vi "FixStyle.vi"(11 "Control in":refnum<class "Control.lvclass">) -> (3 "Control out":refnum<class "Control.lvclass">)   [LabVIEW 2014, in "Control.lvclass"]
uses:
  Control.lvclass
  Control.lvclass/Control.ctl
  Generic/Generic.lvclass/Generic.ctl
  Generic/Generic.lvclass
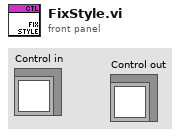
[diagram p1: front panel]
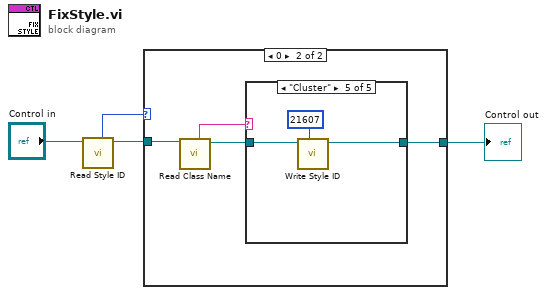
[diagram p0: block diagram]
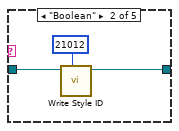
[diagram p4: hidden frame]
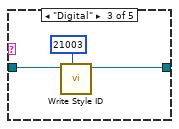
[diagram p5: hidden frame]
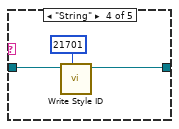
[diagram p6: hidden frame]
diagram:
  n1 = call "Read Style ID.vi"("Control in"="Control in") -> ("Control out"=w2:refnum<class "Control.lvclass">, "Style ID"=w3:u32)  [unwired: 7 in]
  n2 = case shown="0" w3 {
    tunnel: w2 -> [w5 w9]
    tunnel: [w5 w6] -> w1
    frame Default {
    }
    frame 0 {
      n3 = call "Read Class Name.vi"("Generic in"=w9) -> ("Generic out"=w7:refnum<class "Control.lvclass">, "Class Name"=w8:string)  [unwired: 7 in]
      n4 = case shown="\"Cluster\"" w8 {
        tunnel: w7 -> [w10 w13 w16 w19 w22]
        tunnel: [w10 w12 w15 w18 w21] -> w6
        frame Default {
        }
        frame "Boolean" {
          n5 = call "Write Style ID.vi"("Style ID"=u32 21012, "Control in"=w13) -> ("Control out"=w12:refnum<class "Control.lvclass">)  [unwired: 7 in]
        }
        frame "Digital" {
          n6 = call "Write Style ID.vi"("Style ID"=u32 21003, "Control in"=w16) -> ("Control out"=w15:refnum<class "Control.lvclass">)  [unwired: 7 in]
        }
        frame "String" {
          n7 = call "Write Style ID.vi"("Style ID"=u32 21701, "Control in"=w19) -> ("Control out"=w18:refnum<class "Control.lvclass">)  [unwired: 7 in]
        }
        frame "Cluster" {
          n8 = call "Write Style ID.vi"("Style ID"=u32 21607, "Control in"=w22) -> ("Control out"=w21:refnum<class "Control.lvclass">)  [unwired: 7 in]
        }
      }
    }
  }
  "Control out" <- w1
